vi "Cubic Spline Matrices.vi"(8 "Error In":errorcluster, 11 "order":i32) -> (0 "Error Out":errorcluster, 2 "Cubic Spline nxn Matrix Q":T1, 3 "Cubic Spline nxn Matrix M":T1)   [LabVIEW 2021, in "Fits.lvlib"]
uses:
  <vilib>/silver_ctls/ArrayMatrixCluster/Real Matrix NI_Silver.ctl
  <vilib>/Utility/error.llb/Error Cluster From Error Code.vi
  <vilib>/ErrorRing/Error Ring.xnode
  Fits.lvlib
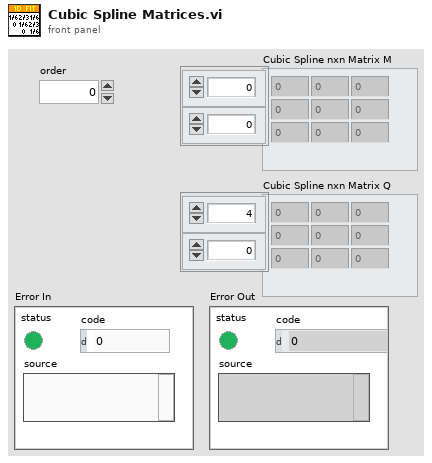
[diagram p1: front panel]
types:
  T1 = typedef "Real Matrix NI_Silver.ctl" = dbl[][]
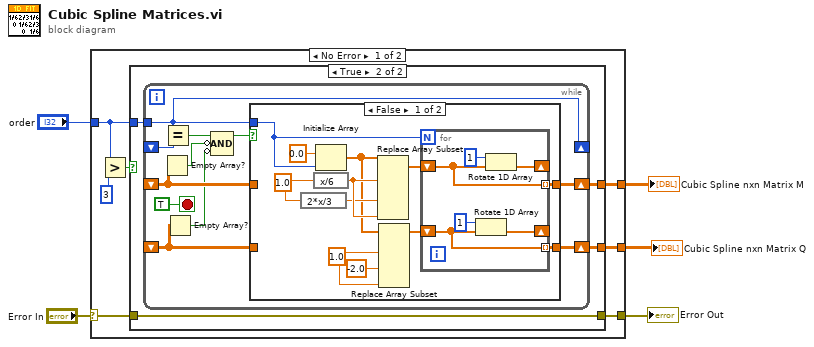
[diagram p0: block diagram]
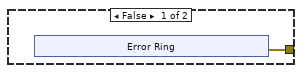
[diagram p2: hidden frame]
diagram:
  n1 = case shown="No Error" "Error In" {
    selector: "Error In" -> [w8 w53]
    tunnel: "order" -> [w11 _]
    tunnel: [w12 _] -> w4
    tunnel: [w7 w53] -> w2
    tunnel: [w6 _] -> w1
    frame No Error {
      n2 = Greater?(x=w11, y=3) -> (0:w9:bool)
      n3 = case shown="True" w9 {
        tunnel: [_ w21] -> w12
        tunnel: w11 -> [_ w20]
        tunnel: w8 -> [_ w19]
        tunnel: [w13 w19] -> w7
        tunnel: [_ w18] -> w6
        frame False {
          n4 = xnode "Error Ring"() -> ("error out"=w13:errorcluster)
        }
        frame True {
          n5 = while {
            tunnel: w20 -> [w29]
            shift-right: [w29] -> _
            shift-left: _ -> [w30]
            shift-right: [w32] -> w21
            shift-left: _ -> [w27]
            shift-right: [w24] -> w18
            shift-left: _ -> [w22]
            stop <- TRUE stop-if-true
            n6 = Empty Array?(array=w27) -> (empty?=w25:bool)
            n7 = Equal?(x=w29, y=w30) -> (x = y?=w28:bool)
            n8 = Empty Array?(array=w22) -> (empty?=w23:bool)
            n9 = Compound Arithmetic op=AND(w28, invert w25, invert w23) -> (w26:bool)
            n10 = case shown="False" w26 {
              tunnel: [w38 w52] -> w32
              tunnel: w29 -> [w39 _]
              tunnel: w27 -> [_ w52]
              tunnel: [w33 w51] -> w24
              tunnel: w22 -> [_ w51]
              frame False {
                w36 = 1.0 ("element")
                w42 = 1.0 ("element")
                n11 = expression code="2*x/3"(w42) -> (w41:dbl)
                n12 = expression code="x/6"(w42) -> (w43:dbl)
                n13 = Initialize Array(0.0 ("element"), w39) -> (w37:dbl[])
                n14 = Replace Array Subset(array=w37, new element #1=w43, new element #2=w41, new element #3=w43) -> (w40:dbl[])  [unwired: 3 in]
                n15 = Replace Array Subset(array=w37, new element #1=w36, new element #2=-2.0 ("new element/subarray"), new element #3=w36) -> (w34:dbl[])  [unwired: 3 in]
                n16 = for {
                  N: w39 -> [_]
                  shift-right: [w49] -> _
                  shift-left: w40 -> [w50]
                  tunnel: [w50] -> w38 mode=indexing
                  shift-right: [w47] -> _
                  shift-left: w34 -> [w45]
                  tunnel: [w45] -> w33 mode=indexing
                  n17 = Rotate 1D Array(1:w45, 2:1 ("n")) -> (0:w47:dbl[])
                  n18 = Rotate 1D Array(1:w50, 2:1 ("n")) -> (0:w49:dbl[])
                }
              }
              frame True {
              }
            }
          }
        }
      }
    }
    frame Error {
    }
  }
  "Cubic Spline nxn Matrix M" <- w4
  "Error Out" <- w2
  "Cubic Spline nxn Matrix Q" <- w1
